vi "kleursensor.vi"(8 "error in (no error)":errorcluster, 10 "High 4":string="—", 11 "Low 4":string="–") -> (0 "error out":errorcluster, 1 "Low 3":u8[](array[numeric]), 2 "Total 2":u32, 3 "High 3":u8[](array[numeric]))   [LabVIEW 2019]
uses:
  <vilib>/myRIO/Instrument Drivers/Onboard IO/I2C/typedefs/I2C Transfer Rate.ctl
  <vilib>/myRIO/Instrument Drivers/Onboard IO/I2C/I2C.lvlib
  <vilib>/myRIO/Instrument Drivers/Onboard IO/I2C/typedefs/I2C User Configuration.ctl
  <vilib>/myRIO/Instrument Drivers/Onboard IO/I2C/typedefs/I2C Configuration.ctl
  <vilib>/myRIO/Common/Instrument Driver Framework/myRIO v1.0/I2C/typedefs/I2C Channels Enum.ctl
  <vilib>/myRIO/Common/Instrument Driver Framework/Utilities/typedefs/Generic FPGA Reference.ctl
  <vilib>/myRIO/Common/Instrument Driver Framework/Utilities/typedefs/myRIO v1.0 Reference.ctl
  <vilib>/myRIO/Common/Instrument Driver Framework/Utilities/typedefs/Hardware Version Enum.ctl
  <vilib>/myRIO/Common/Instrument Driver Framework/Utilities/typedefs/myRIO Generic Hardware Reference.ctl
  <vilib>/myRIO/Instrument Drivers/Onboard IO/I2C/typedefs/I2C Reference.ctl
  <vilib>/myRIO/Instrument Drivers/Onboard IO/I2C/vis/Configure.vi
  <vilib>/myRIO/Instrument Drivers/Onboard IO/I2C/vis/Write Read.vi
  <vilib>/userDefined/High Color/nirio_resource_hc.ctl
  <vilib>/myRIO/Common/Instrument Driver Framework/myRIO v1.0/I2C/vis/myRIO v1.1 Open I2C.vi
  <vilib>/myRIO/Instrument Drivers/Onboard IO/I2C/vis/myRIO I2C Open.xnode
  <vilib>/myRIO/Common/Instrument Driver Framework/Utilities/vis/Is FPGA Ref Available.vi
  <vilib>/myRIO/Express VI/Onboard IO/I2C/I2C Express VI.xnode
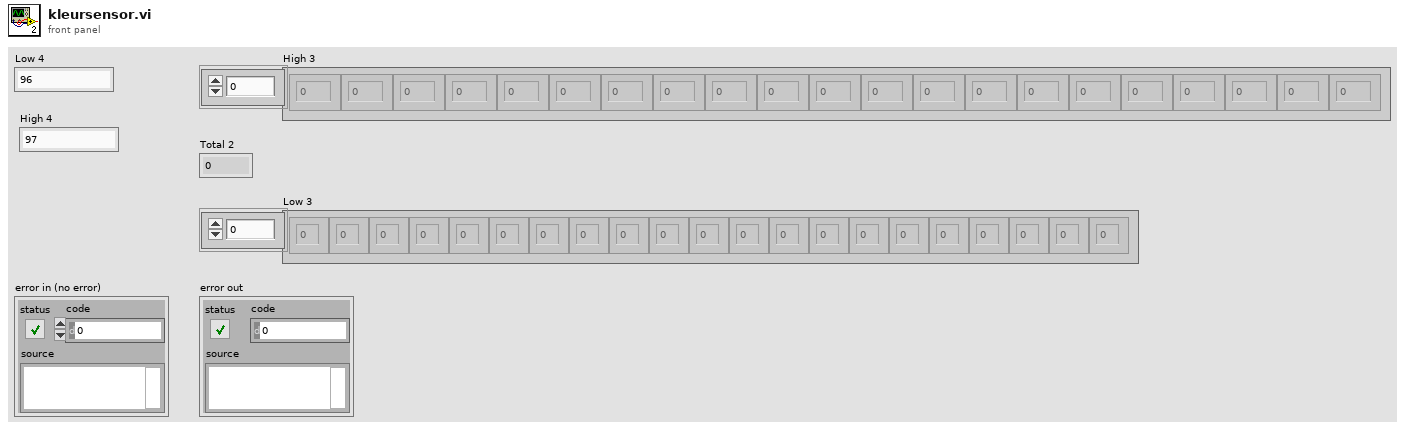
[diagram p1: front panel]
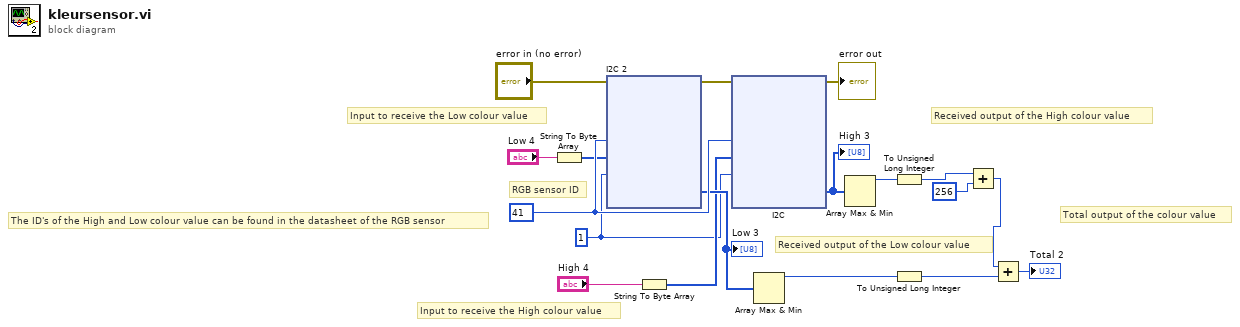
[diagram p0: block diagram]
diagram:
  w18 = 41 ("Numeric")
  w8 = u32 1 ("Byte Count")
  # "Total output of the colour value"
  # "Received output of the Low colour value"
  # "Received output of the High colour value"
  # "The ID's of the High and Low colour value can be found in the datasheet of the RGB sensor"
  # "Input to receive the Low colour value"
  # "Input to receive the High colour value"
  # "RGB sensor ID"
  n1 = String To Byte Array(string="Low 4") -> (unsigned byte array=w9:u8[])
  n2 = xnode "I2C 2"("Slave Address (7-bit)"=w18, "Bytes to Write"=w9, "Byte Count"=w8, "error in (no error)"="error in (no error)") -> ("Bytes Read"=w12:u8[], "error out"=w7:errorcluster)
  "Low 3" <- w12
  n3 = String To Byte Array(string="High 4") -> (unsigned byte array=w10:u8[])
  n4 = xnode "I2C"("Slave Address (7-bit)"=w18, "Bytes to Write"=w10, "Byte Count"=w8, "error in (no error)"=w7) -> ("Bytes Read"=w13:u8[], "error out"=→"error out":errorcluster)
  "High 3" <- w13
  n5 = Array Max & Min(array=w12) -> (max value=w16:u8)  [unwired: 3 out]
  n6 = Array Max & Min(array=w13) -> (max value=w15:u8)  [unwired: 3 out]
  n7 = To Unsigned Long Integer(number=w15) -> (unsigned 32bit integer=w2:u32)
  n8 = To Unsigned Long Integer(number=w16) -> (unsigned 32bit integer=w17:u32)
  n9 = Add(x=w2, y=u32 256) -> (x+y=w1:u32)
  n10 = Add(x=w1, y=w17) -> (x+y=→"Total 2":u32)
